vi "PID with Diff Drive FF.vi"(5 "output range":cluster{"output high":dbl, "output low":dbl}={"output high"=1.0, "output low"=-1.0}, 6 "reinitialize? (F)":bool, 7 "Feed Forward Constants":T1, 8 "dt (s)":dbl=0.01, 9 "Acceleration (0)":dbl, 10 "Velocity":dbl format="%#_13g", 11 "Velocity Reference":dbl format="%#_13g") -> (3 "Output":dbl)   [LabVIEW 2019]
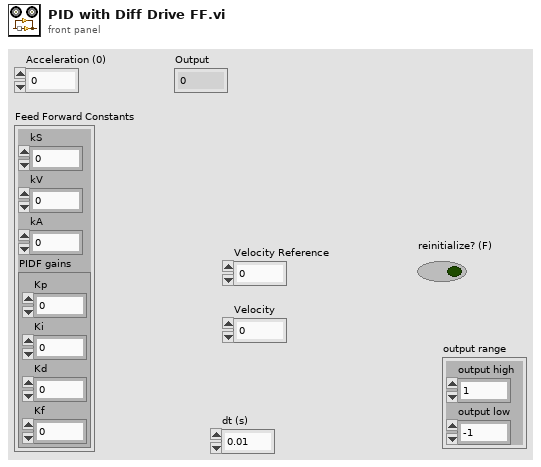
[diagram p1: front panel]
types:
  T1 = cluster{"kS":dbl, "kV":dbl, "kA":dbl, "PIDF gains":cluster{"Kp":dbl, "Ki":dbl, "Kd":dbl, "Kf":dbl}}
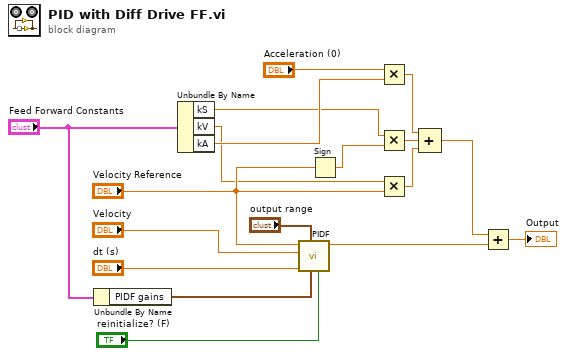
[diagram p0: block diagram]
diagram:
  n1 = Unbundle By Name("Feed Forward Constants") -> ("PIDF gains"=w17:cluster{"Kp":dbl, "Ki":dbl, "Kd":dbl, "Kf":dbl})
  n2 = Unbundle By Name("Feed Forward Constants") -> ("kS"=w4:dbl, "kV"=w5:dbl, "kA"=w8:dbl)
  n3 = call "PIDF.vi"("reinitialize? (F)"="reinitialize? (F)", "PIDF gains"=w17, "output range"="output range", "dt (s)"="dt (s)", "process variable"="Velocity", "setpoint"="Velocity Reference") -> ("output"=w13:dbl)  [unwired: 3 in, 2 out]
  n4 = Sign(1:"Velocity Reference") -> (0:w3:dbl)
  n5 = Multiply(x="Acceleration (0)", y=w8) -> (x*y=w9:dbl)
  n6 = Multiply(x=w4, y=w3) -> (x*y=w11:dbl)
  n7 = Multiply(x=w5, y="Velocity Reference") -> (x*y=w10:dbl)
  n8 = Compound Arithmetic op=ADD(w9, w11, w10) -> (w12:dbl)
  n9 = Add(x=w12, y=w13) -> (x+y=→"Output":dbl)
